vi "PolStop-C.vi"(3 "error in (no error)":errorcluster, 4 "Sync In? (F)":bool, 5 "VISA resource name":refnum<visa-resource-name>) -> (0 "error out":errorcluster, 2 "VISA resource name out":refnum<visa-resource-name>)   [LabVIEW 2012]
doc: "Stops Polhemus output. \n\nNormally sends a 'c' command to stop continous output.\n\nIf externally syncing, sends a y0 command. IMPORTANT: Polhemus must recieve one more sync pulse for this to take effect."
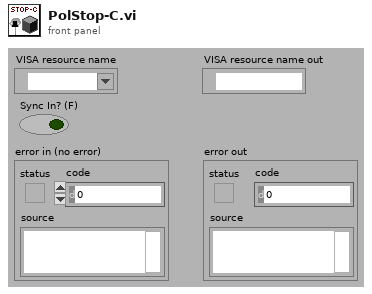
[diagram p1: front panel]
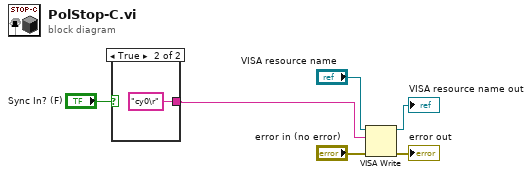
[diagram p0: block diagram]
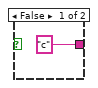
[diagram p2: hidden frame]
diagram:
  n1 = case shown="True" "Sync In? (F)" {
    tunnel: ["c" ("write buffer") "cy0\r" ("write buffer")] -> w1
    frame False {
    }
    frame True {
    }
  }
  n2 = VISA Write(VISA resource name="VISA resource name", write buffer=w1, error in (no error)="error in (no error)") -> (VISA resource name out=→"VISA resource name out":refnum<visa-resource-name>, error out=→"error out":errorcluster)  [unwired: 1 out]
